vi "Edit_Raw_DF_Header.vi"(0 "Selected files":path[](array[path])) -> ()   [LabVIEW 2017]
uses:
  Controls/File_Selector_Type.ctl
panel:
  in  "Variable names to add by hand":string[](array[string])
  in  "Variable values to add by hand":string[](array[string])
  out "No of Unfound files":i32
  out "Unfound Files":path[](array[path])
  out "File Number":i32
  out "Current case":string
  out "Currently Editting":path
  out "Summary values":string[](array[string])
  in  "New Variable values":string[](array[string])
  in  "Setup Information":i32[](listbox)
  in  "Variable names to Edit":string[](array[string])
  in  "OK":bool
  out "No of Files":i32
  in  "Previous Choice":path
  in  "Search String":string
  in  "At Dialog Prompt for Editting Raw data files":T1
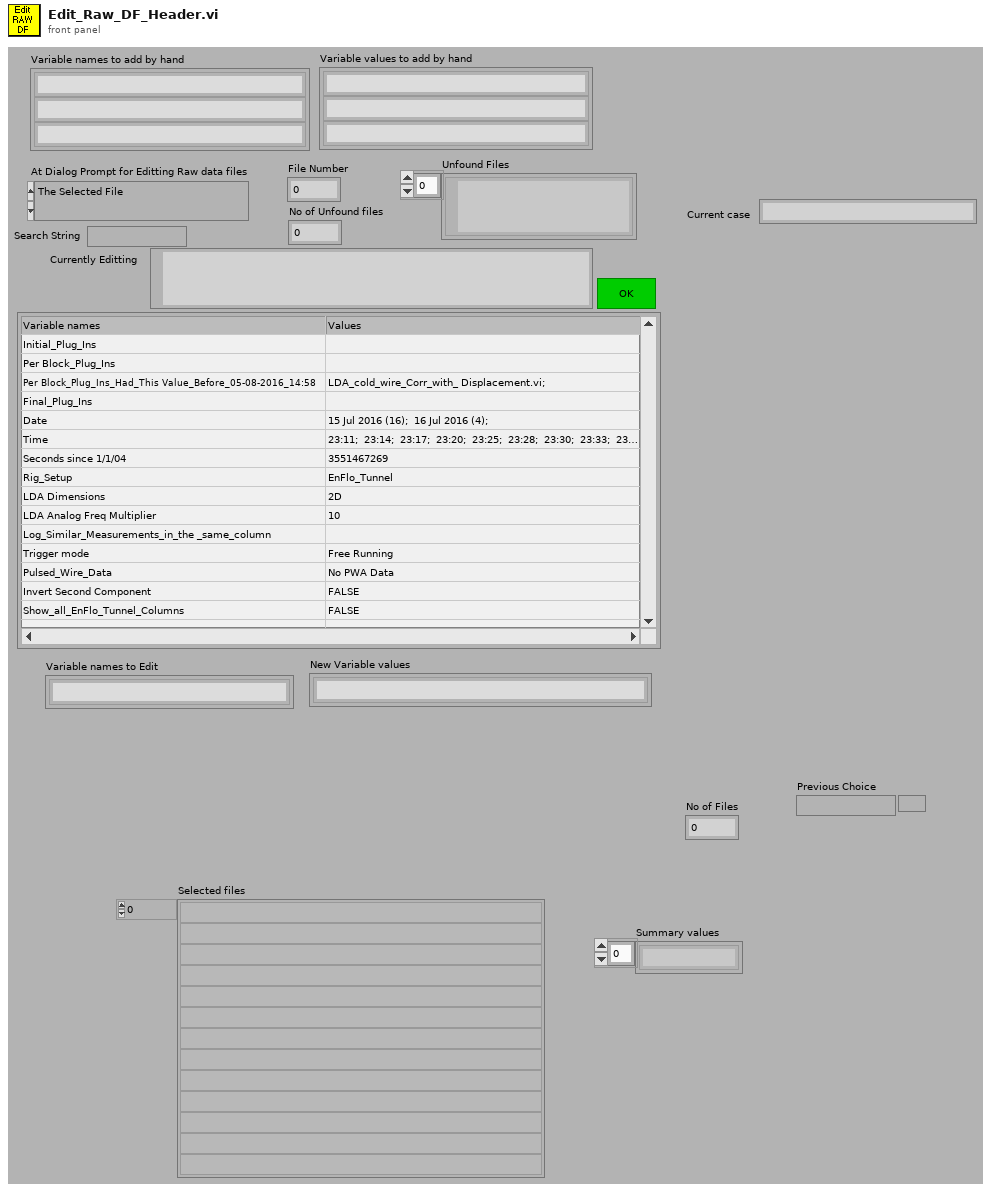
[diagram p1: front panel]
types:
  T1 = typedef "File_Selector_Type.ctl" = enum16{"The Selected File", "The Selected Folder", "Files containing the search string in the selected folder", "All files listed in selected file"}
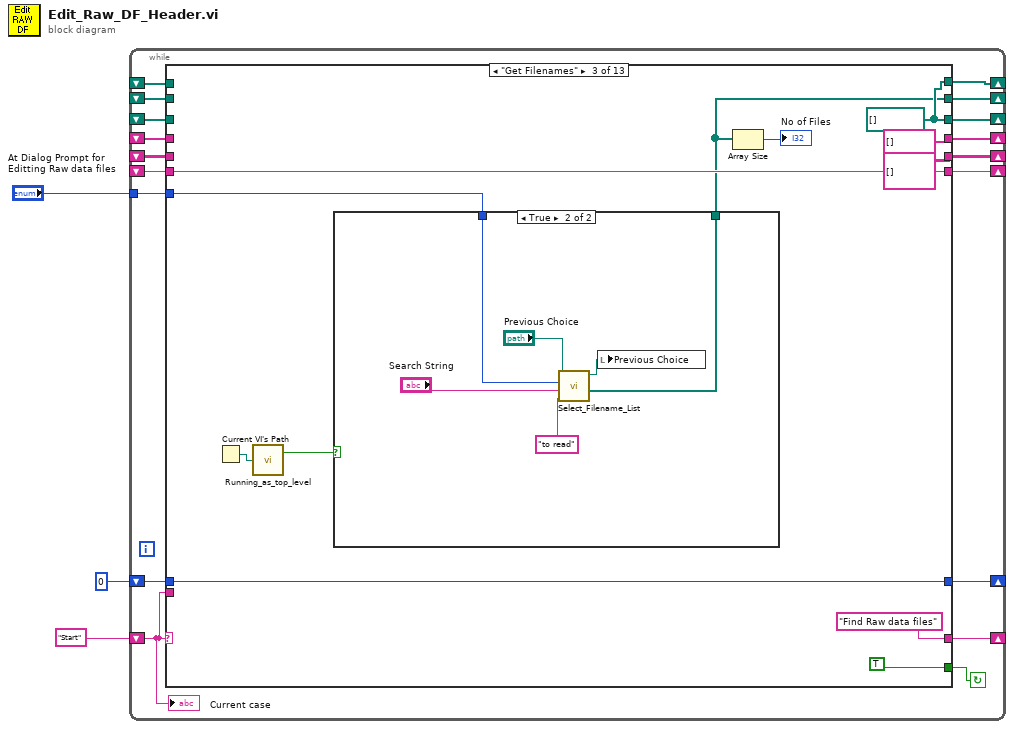
[diagram p0: block diagram]
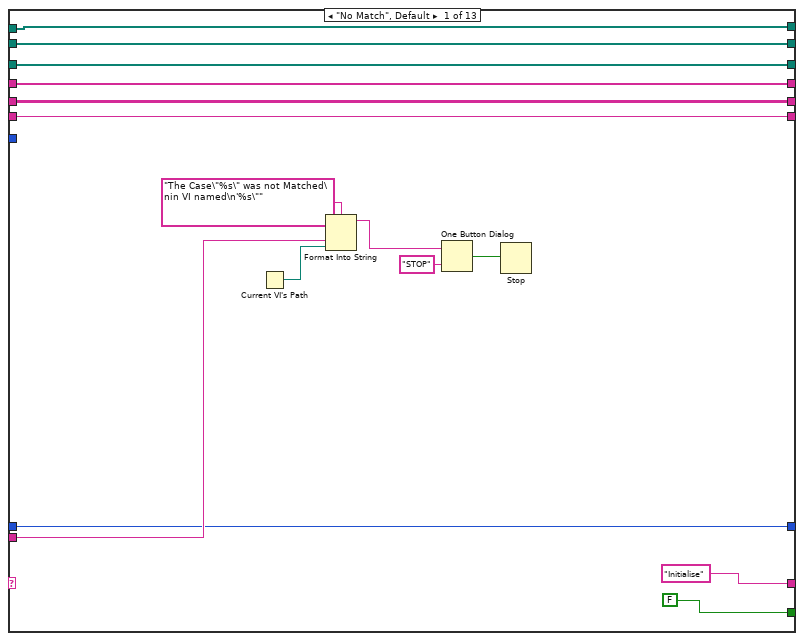
[diagram p2: hidden frame]
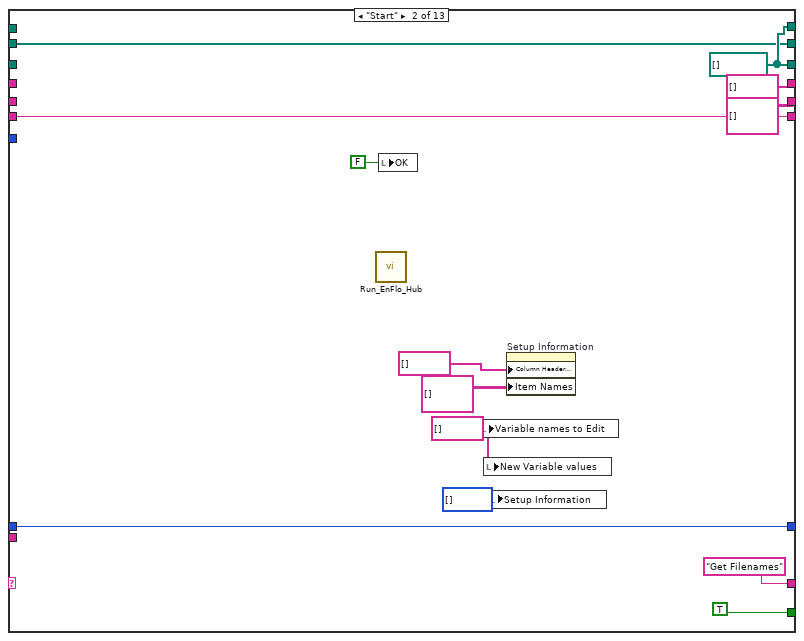
[diagram p3: hidden frame]
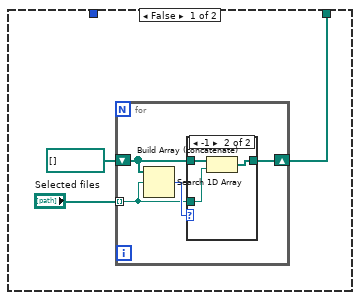
[diagram p4: hidden frame]
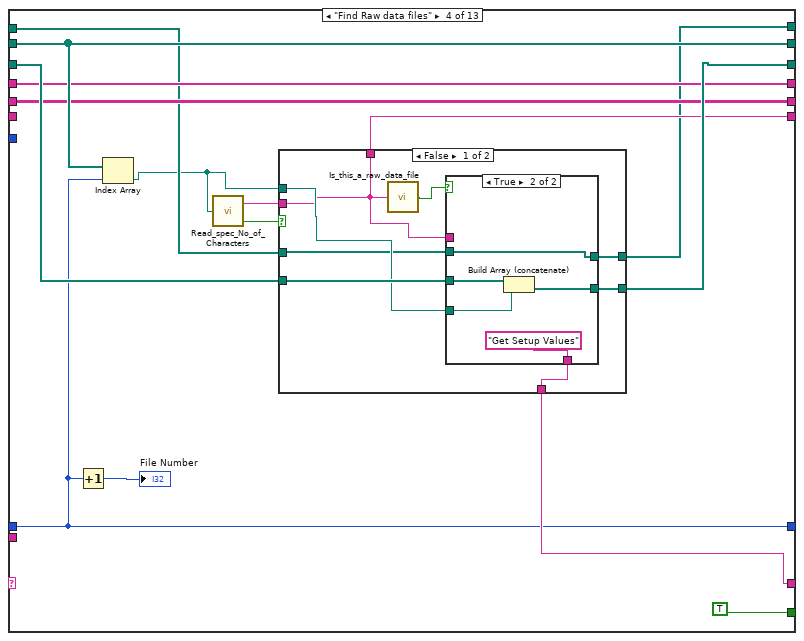
[diagram p6: hidden frame]
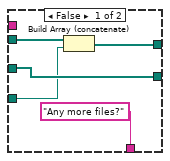
[diagram p7: hidden frame]
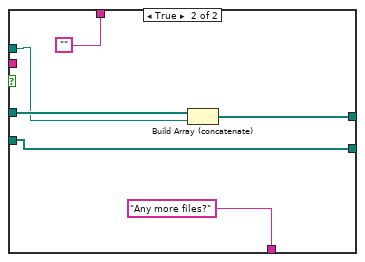
[diagram p8: hidden frame]
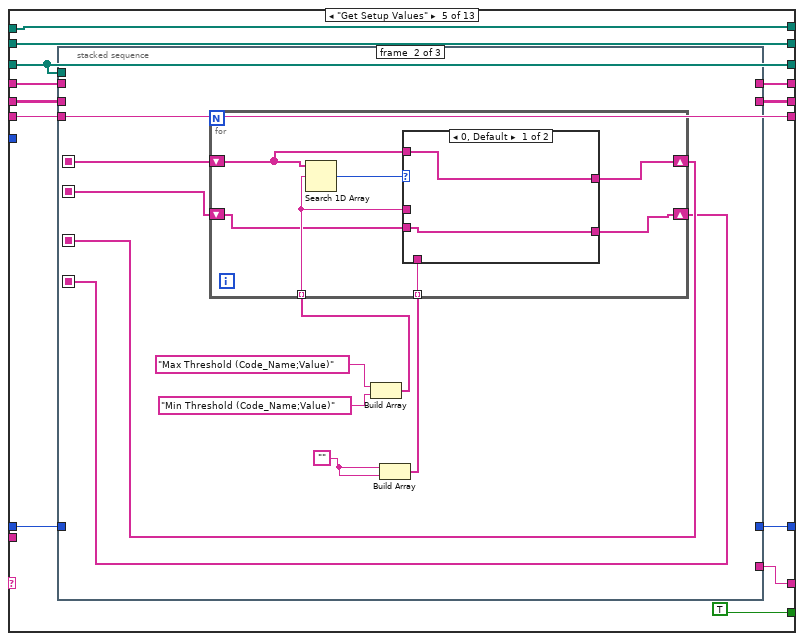
[diagram p9: hidden frame]
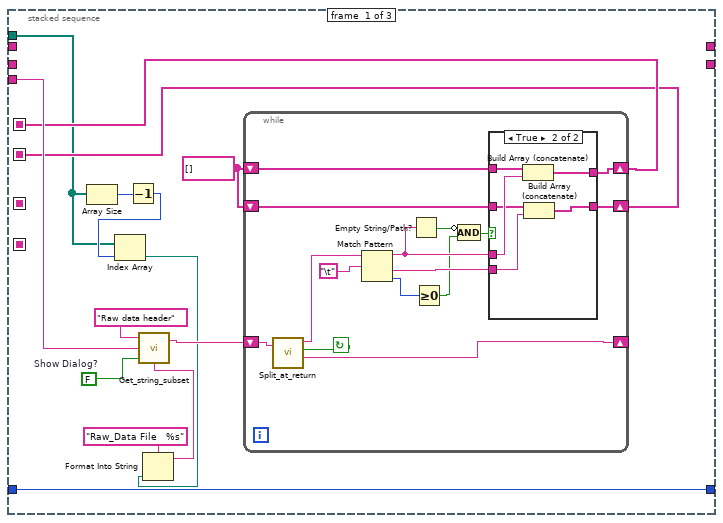
[diagram p10: hidden frame]
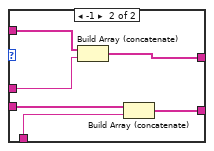
[diagram p12: hidden frame]
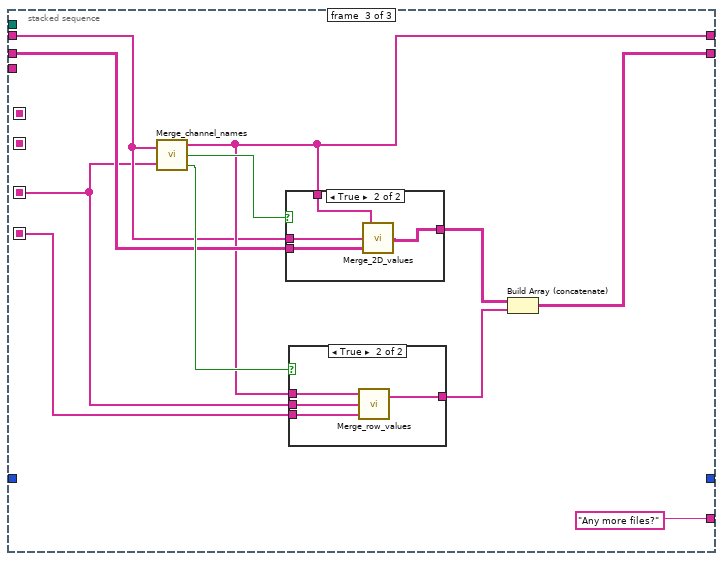
[diagram p13: hidden frame]
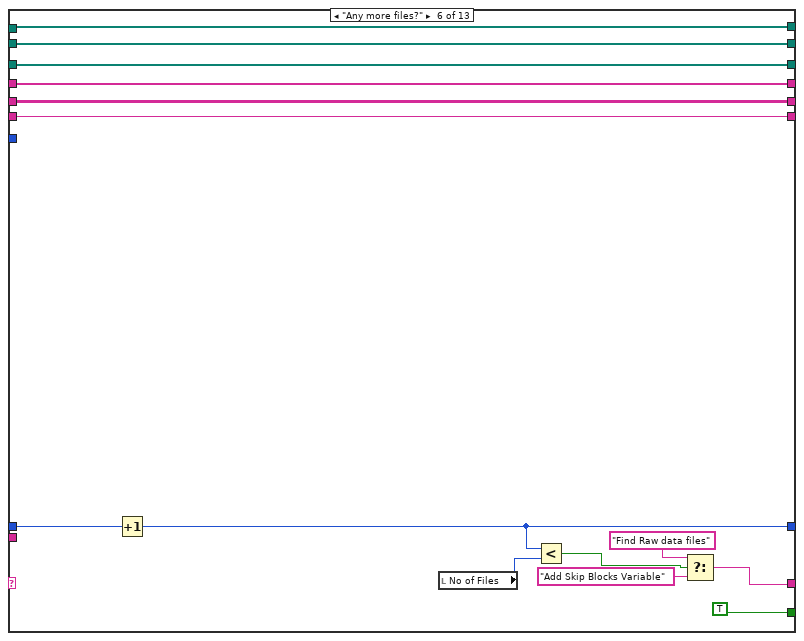
[diagram p16: hidden frame]
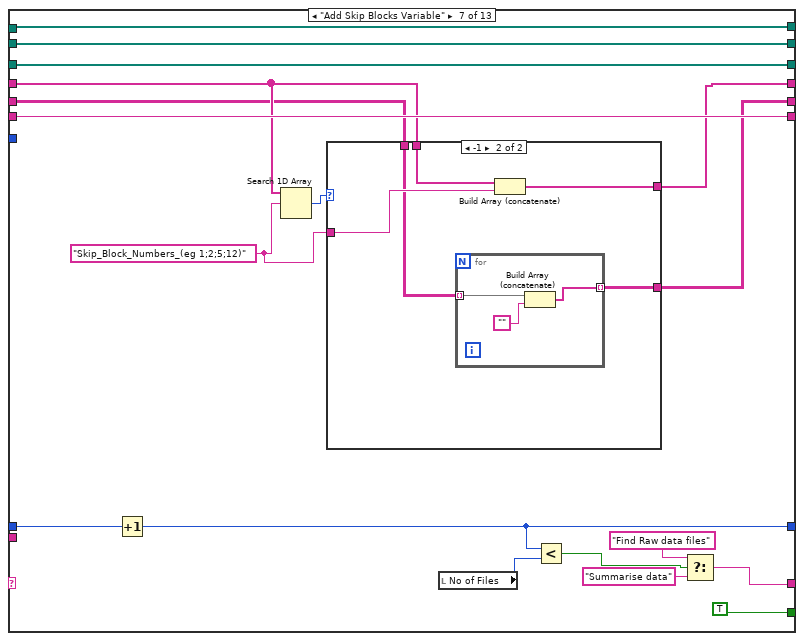
[diagram p17: hidden frame]
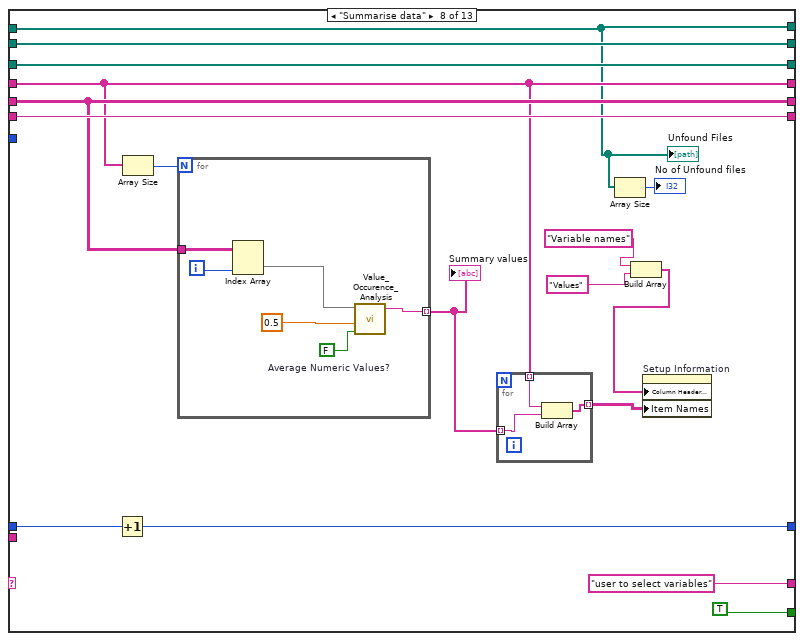
[diagram p19: hidden frame]
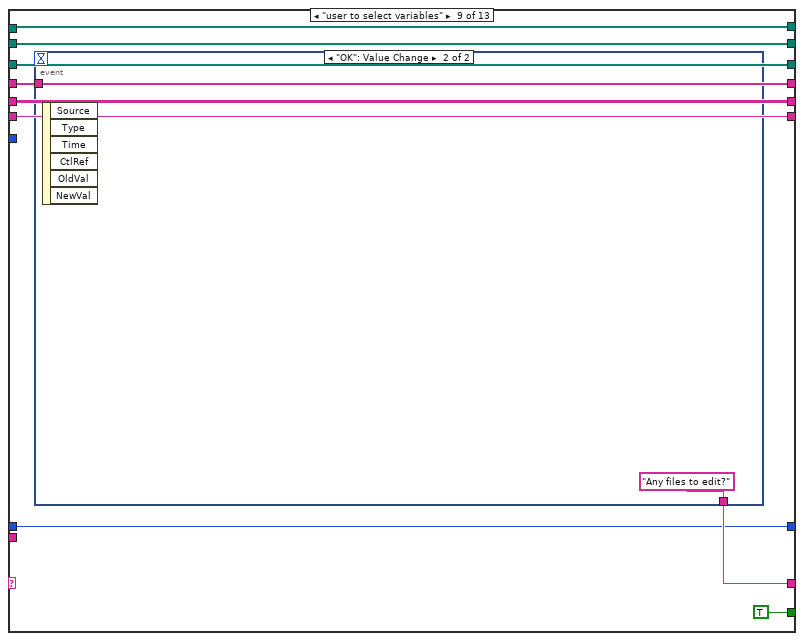
[diagram p20: hidden frame]
diagram:
  n1 = while {
    shift-left: "Start" -> [w19]
    shift-right: [w20] -> _
    shift-right: [w17] -> _
    shift-left: _ -> [w18]
    tunnel: "At Dialog Prompt for Editting Raw data files" -> [w16]
    shift-right: [w7] -> _
    shift-left: 0 -> [w13]
    shift-right: [w15] -> _
    shift-left: _ -> [w14]
    shift-right: [w12] -> _
    shift-left: _ -> [w11]
    shift-right: [w9] -> _
    shift-left: _ -> [w10]
    shift-right: [w8] -> _
    shift-left: _ -> [w6]
    shift-right: [w4] -> _
    shift-left: _ -> [w5]
    stop <- w21 continue-if-true
    n2 = case shown="\"Get Filenames\"" w19 {
      tunnel: [FALSE TRUE TRUE TRUE TRUE TRUE TRUE TRUE TRUE w323 w362 TRUE ("T button?") FALSE ("T button?")] -> w21
      tunnel: ["Initialise" "Get Filenames" "Find Raw data files" w86 w125 w217 w236 "user to select variables" w282 "Shall I edit the data files?" "Edit Raw data files" "End" "End"] -> w20
      tunnel: w19 -> [w31 _ _ _ _ _ _ _ _ _ _ _ _]
      tunnel: w18 -> [w28 w37 _ w90 w128 w224 w242 w269 w288 w336 w372 w383 w398]
      tunnel: [w28 w37 w50 w90 w128 w224 w242 w269 w288 w336 w372 w383 w398] -> w17
      tunnel: w16 -> [_ _ w60 _ _ _ _ _ _ _ _ _ _]
      tunnel: w14 -> [w27 _ _ w92 w118 w216 w235 w266 w287 w333 w366 w376 w392]
      tunnel: [w27 w38 w53 w91 w118 w216 w235 w266 w287 w333 w366 w376 w392] -> w15
      tunnel: w13 -> [w23 w44 w54 w85 w127 w222 w241 w268 w281 w335 w367 w378 w393]
      tunnel: [w26 string[] [] ("Merged Channels") string[] [] ("Merged Channels") w89 w123 w212 w230 w262 w283 w321 w369 w380 w395] -> w12
      tunnel: w11 -> [w26 _ _ w89 w120 w212 w231 w262 w283 w321 w369 w380 w395]
      tunnel: w10 -> [w25 _ _ w88 w122 w223 w227 w264 w285 w331 w370 w381 w396]
      tunnel: [w25 string[][] [] string[][] [] w88 w121 w223 w226 w264 w285 w331 w370 w381 w396] -> w9
      tunnel: [w24 w47 w57 w87 w124 w215 w234 w265 w286 w332 w371 w382 w397] -> w8
      tunnel: [w23 w44 w54 w85 w126 w221 w240 w267 w281 w334 w367 w378 w393] -> w7
      tunnel: w6 -> [w24 w47 w57 _ w124 w215 w234 w265 w286 w332 w371 w382 w397]
      tunnel: w5 -> [w22 _ _ w84 w119 w213 w232 w255 w280 w322 w361 w373 w388]
      tunnel: [w22 w38 w53 w83 w119 w213 w232 w255 w280 w322 w361 w373 w388] -> w4
      frame "No Match", Default {
        n3 = Current VI's Path() -> (path=w30:path)
        n4 = Format Into String(format string="The Case\"%s\" was not Matched\nin VI named\n'%s\"" ("Format String"), w31, w30) -> (resulting string=w34:string)  [unwired: 2 in, 1 out]
        n5 = One Button Dialog(message=w34, button name ("OK")="STOP") -> (true=w32:bool)
        n6 = Stop(stop? (T)=w32) -> ()
      }
      frame "Start" {
        w43 = string[] [] ("Variable names to Edit")
        w38 = path[] []
        n7 = call "Run_EnFlo_Hub.vi"() -> ()  [unwired: 1 in, 7 out]
        n8 = local write "OK"(FALSE ("OK")) -> ()
        n9 = local write "Variable names to Edit"(w43) -> ()
        n10 = local write "New Variable values"(w43) -> ()
        n11 = local write "Setup Information"(i32[] [] ("Setup Information")) -> ()
        n12 = property on="Setup Information" class="MCListbox (strict)"("Column Header Strings[]"=string[] [] ("Column Header Strings"), "Item Names"=string[][] []) -> ()  [unwired: 2 in, 2 out]
      }
      frame "Get Filenames" {
        w53 = path[] []
        n13 = Current VI's Path() -> (path=w52:path)
        n14 = call "Running_as_top_level.vi"("Vi path name"=w52) -> ("Top Level"=w51:bool)  [unwired: 1 out]
        n15 = case shown="True" w51 {
          tunnel: w60 -> [_ w78]
          tunnel: [w62 w73] -> w50
          frame False {
            n16 = for {
              shift-right: [w65] -> w62
              shift-left: path[] [] -> [w66]
              tunnel: "Selected files" -> [w67] mode=indexing
              n17 = Search 1D Array(1D array=w66, element=w67) -> (index of element=w68:i32)  [unwired: 1 in]
              n18 = case shown="-1" w68 {
                tunnel: w67 -> [_ w72]
                tunnel: w66 -> [w69 w71]
                tunnel: [w69 w70] -> w65
                frame Default {
                }
                frame -1 {
                  n19 = Build Array (concatenate)(w71, w72) -> (w70:path[])
                }
              }
            }
          }
          frame True {
            n20 = call "Select_Filename_List.vi"("File Type"="to read", "Search String"="Search String", "At Dialog Prompt Post Process"=w78, "Previous Choice"="Previous Choice") -> ("Selected files"=w73:path[], "Choosen path"=w74:path)  [unwired: 1 in, 2 out]
            n21 = local write "Previous Choice"(w74) -> ()
          }
        }
        n22 = Array Size(array=w50) -> (size(s)=→"No of Files":i32)
      }
      frame "Find Raw data files" {
        n23 = Increment(x=w85) -> (x+1=→"File Number":i32)
        n24 = Index Array(array=w90, index=w85) -> (element=w82:path)
        n25 = call "Read_spec_No_of_Characters.vi"("Filename"=w82) -> ("character string"=w80:string, "Error?"=w81:bool)
        n26 = case shown="False" w81 {
          tunnel: w92 -> [w101 w117]
          tunnel: [w100 w117] -> w91
          tunnel: w82 -> [w98 w113]
          tunnel: [w94 ""] -> w87
          tunnel: [w97 "Any more files?"] -> w86
          tunnel: w84 -> [w96 w114]
          tunnel: [w95 w112] -> w83
          tunnel: w80 -> [w94 _]
          frame False {
            n27 = call "Is_this_a_raw_data_file.vi"("character string"=w94) -> ("Raw Dat File?"=w99:bool)  [unwired: 2 out]
            n28 = case shown="True" w99 {
              tunnel: w101 -> [w106 w111]
              tunnel: w98 -> [w102 w110]
              tunnel: [w106 w109] -> w100
              tunnel: w94 -> [_ _]
              tunnel: ["Any more files?" "Get Setup Values"] -> w97
              tunnel: w96 -> [w104 w107]
              tunnel: [w103 w107] -> w95
              frame False {
                n29 = Build Array (concatenate)(w104, w102) -> (w103:path[])
              }
              frame True {
                n30 = Build Array (concatenate)(w111, w110) -> (w109:path[])
              }
            }
          }
          frame True {
            n31 = Build Array (concatenate)(w114, w113) -> (w112:path[])
          }
        }
      }
      frame "Get Setup Values" {
        n32 = stacked-sequence {
          seq-local: [w137 _ _] -> [_ w175 _]
          seq-local: [w136 _ _] -> [_ w171 _]
          seq-local: [_ w168 _] -> [_ _ w192]
          seq-local: [_ w167 _] -> [_ _ w191]
          tunnel: w127 -> [w140 _ _]
          tunnel: [w140 _ _] -> w126
          tunnel: [_ _ "Any more files?"] -> w125
          tunnel: w124 -> [w141 _ _]
          tunnel: w120 -> [_ _ w193]
          tunnel: [_ _ w195] -> w123
          tunnel: w122 -> [_ _ w199]
          tunnel: [_ _ w196] -> w121
          tunnel: w118 -> [w131 _ _]
          frame #0 {
            w138 = string[] []
            w143 = FALSE  # Show Dialog?
            n33 = Array Size(array=w131) -> (size(s)=w133:i32)
            n34 = Decrement(x=w133) -> (x-1=w132:i32)
            n35 = Index Array(array=w131, index=w132) -> (element=w130:path)
            n36 = Format Into String(format string="Raw_Data File   %s", w130) -> (resulting string=w134:string)  [unwired: 2 in, 1 out]
            n37 = call "Get_string_subset.vi"("String Name"=w134, "Show Dialog?"=w143, "String to split"=w141, "File Label"="Raw data header") -> ("Output string"=w139:string)  [unwired: 1 out]
            n38 = while {
              shift-right: [w157] -> _
              shift-left: w139 -> [w158]
              shift-right: [w151] -> w137
              shift-left: w138 -> [w152]
              shift-right: [w149] -> w136
              shift-left: w138 -> [w150]
              stop <- w156 continue-if-true
              n39 = call "Split_at_return.vi"("String"=w158) -> ("before substring"=w154:string, "Matched?"=w156:bool, "after substring"=w157:string)  [unwired: 1 in, 1 out]
              n40 = Match Pattern(string=w154, regular expression="\t") -> (before substring=w147:string, after substring=w148:string, offset past match=w153:i32)  [unwired: 2 out]
              n41 = Empty String/Path?(string/path=w147) -> (empty?=w146:bool)
              n42 = Greater Or Equal To 0?(x=w153) -> (x >= 0?=w144:bool)
              n43 = Compound Arithmetic op=AND(invert w146, w144) -> (w145:bool)
              n44 = case shown="True" w145 {
                tunnel: w152 -> [w160 w166]
                tunnel: w147 -> [_ w165]
                tunnel: [w160 w164] -> w151
                tunnel: w150 -> [w159 w163]
                tunnel: [w159 w162] -> w149
                tunnel: w148 -> [_ w161]
                frame False {
                }
                frame True {
                  n45 = Build Array (concatenate)(w166, w165) -> (w164:string[])
                  n46 = Build Array (concatenate)(w163, w161) -> (w162:string[])
                }
              }
            }
          }
          frame #1 {
            w169 = ""
            n47 = Build Array("Max Threshold (Code_Name;Value)", "Min Threshold (Code_Name;Value)") -> (w172:string[])
            n48 = Build Array(w169, w169) -> (w170:string[])
            n49 = for {
              shift-right: [w179] -> w168
              shift-left: w175 -> [w181]
              tunnel: w172 -> [w180] mode=indexing
              shift-right: [w176] -> w167
              shift-left: w171 -> [w178]
              tunnel: w170 -> [w177] mode=indexing
              n50 = Search 1D Array(1D array=w181, element=w180) -> (index of element=w182:i32)  [unwired: 1 in]
              n51 = case shown="0, Default" w182 {
                tunnel: w181 -> [w184 w190]
                tunnel: w180 -> [_ w189]
                tunnel: [w184 w188] -> w179
                tunnel: w178 -> [w183 w187]
                tunnel: w177 -> [_ w186]
                tunnel: [w183 w185] -> w176
                frame 0, Default {
                }
                frame -1 {
                  n52 = Build Array (concatenate)(w190, w189) -> (w188:string[])
                  n53 = Build Array (concatenate)(w187, w186) -> (w185:string[])
                }
              }
            }
          }
          frame #2 {
            n54 = call "Merge_channel_names.vi"("Preferred Channel array"=w193, "Channel array"=w192) -> ("Merged Channels"=w195:string[], "Preferred Channels Changed?"=w200:bool, "Channel Array Changed?"=w201:bool)
            n55 = case shown="True" w200 {
              tunnel: w199 -> [w207 w209]
              tunnel: w193 -> [_ w211]
              tunnel: [w207 w208] -> w198
              tunnel: w195 -> [_ w210]
              frame False {
              }
              frame True {
                n56 = call "Merge_2D_values.vi"("Values In"=w209, "Present Channels"=w211, "Desired Channels"=w210) -> ("Values Out"=w208:string[][])
              }
            }
            n57 = case shown="True" w201 {
              tunnel: [w202 w206] -> w197
              tunnel: w195 -> [_ w205]
              tunnel: w192 -> [_ w204]
              tunnel: w191 -> [w202 w203]
              frame False {
              }
              frame True {
                n58 = call "Merge_row_values.vi"("Present Row values"=w203, "Present Channels"=w204, "Desired Channels"=w205) -> ("Desired Row values"=w206:string[])  [unwired: 1 out]
              }
            }
            n59 = Build Array (concatenate)(w198, w197) -> (w196:string[][])
          }
        }
      }
      frame "Any more files?" {
        n60 = Increment(x=w222) -> (x+1=w221:i32)
        n61 = local read "No of Files"() -> (w220:i32)
        n62 = Less?(x=w221, y=w220) -> (x < y?=w219:bool)
        n63 = Select(t="Find Raw data files", s=w219, f="Add Skip Blocks Variable") -> (s? t:f=w217:string)
      }
      frame "Add Skip Blocks Variable" {
        w229 = "Skip_Block_Numbers_(eg 1;2;5;12)" ("Variable name")
        n64 = Increment(x=w241) -> (x+1=w240:i32)
        n65 = Search 1D Array(1D array=w231, element=w229) -> (index of element=w228:i32)  [unwired: 1 out]
        n66 = case shown="-1" w228 {
          tunnel: w231 -> [w245 w250]
          tunnel: w229 -> [_ w249]
          tunnel: [w245 w248] -> w230
          tunnel: w227 -> [w244 w247]
          tunnel: [w244 w246] -> w226
          frame 0, Default {
          }
          frame -1 {
            n67 = for {
              tunnel: w247 -> [w252] mode=indexing
              tunnel: [w251] -> w246 mode=indexing
              n68 = Build Array (concatenate)(w252, "") -> (w251:string[])
            }
            n69 = Build Array (concatenate)(w250, w249) -> (w248:string[])
          }
        }
        n70 = local read "No of Files"() -> (w239:i32)
        n71 = Less?(x=w240, y=w239) -> (x < y?=w238:bool)
        n72 = Select(t="Find Raw data files", s=w238, f="Summarise data") -> (s? t:f=w236:string)
      }
      frame "Summarise data" {
        n73 = Increment(x=w268) -> (x+1=w267:i32)
        n74 = Array Size(array=w262) -> (size(s)=w263:i32)
        n75 = for {
          N: w263 -> [_]
          tunnel: w264 -> [w278]
          tunnel: [w274] -> w261 mode=indexing
          i -> [w279]
          w275 = FALSE  # Average Numeric Values?
          n76 = Index Array(array=w278, index (col)=w279) -> (element=w277:string[])  [unwired: 1 in]
          n77 = call "Value_Occurence_Analysis.vi"("Average Numeric Values?"=w275, "Tolerance"=0.5, "String Array"=w277) -> ("Output String"=w274:string)  [unwired: 1 in, 2 out]
        }
        "Summary values" <- w261
        n78 = for {
          tunnel: w262 -> [w272] mode=indexing
          tunnel: w261 -> [w273] mode=indexing
          tunnel: [w271] -> w257 mode=indexing
          n79 = Build Array(w272, w273) -> (w271:string[])
        }
        n80 = Array Size(array=w255) -> (size(s)=→"No of Unfound files":i32)
        n81 = Build Array("Variable names", "Values") -> (w256:string[])
        n82 = property on="Setup Information" class="MCListbox (strict)"("Column Header Strings[]"=w256, "Item Names"=w257) -> ()  [unwired: 2 in, 2 out]
        "Unfound Files" <- w255
      }
      frame "user to select variables" {
        n83 = event shown="[1] \"OK\": Value Change" {
          selector: _ -> [_ _]
          dyn-events: _ -> [_ _]
          timeout: _ -> [_ _]
          tunnel: w283 -> [w297 _]
          tunnel: ["user to select variables" "Any files to edit?"] -> w282
          event "Setup Information": Value Change {
            n84 = event-data() -> ("NewVal"=w298:i32[])  [unwired: 6 out]
            n85 = local read "Summary values"() -> (w296:string[])
            n86 = for {
              tunnel: w298 -> [w304] mode=indexing
              tunnel: w297 -> [w307]
              tunnel: "Variable names to Edit" -> [w306]
              tunnel: [w305] -> w290 mode=indexing
              tunnel: w296 -> [w303]
              tunnel: [w302] -> w295 mode=indexing
              tunnel: "New Variable values" -> [w300]
              tunnel: [w299] -> w292
              i -> [w299]
              n87 = Index Array(array=w307, index=w304) -> (element=w305:string)
              n88 = Search 1D Array(1D array=w306, element=w305) -> (index of element=w301:i32)  [unwired: 1 out]
              n89 = case shown="-1" w301 {
                tunnel: w304 -> [_ w313]
                tunnel: w303 -> [_ w312]
                tunnel: [w308 w311] -> w302
                tunnel: w301 -> [w310 _]
                tunnel: w300 -> [w309 _]
                frame 0, Default {
                  n90 = Index Array(array=w309, index=w310) -> (element=w308:string)
                }
                frame -1 {
                  n91 = Index Array(array=w312, index=w313) -> (element=w311:string)
                }
              }
            }
            n92 = Increment(x=w292) -> (x+1=w291:i32)
            n93 = local write "New Variable values"(w295) -> ()
            n94 = local write "Variable names to Edit"(w290) -> ()
            n95 = property on="Variable names to Edit" class="Arr (strict)"("Number of Rows"=w291) -> ()  [unwired: 2 in, 2 out]
            n96 = property on="New Variable values" class="Arr (strict)"("Number of Rows"=w291) -> ()  [unwired: 2 in, 2 out]
          }
          event "OK": Value Change {
            n97 = event-data() -> ()  [unwired: 7 out]
          }
        }
      }
      frame "Any files to edit?" {
        w327 = string[] []
        n98 = local read "New Variable values"() -> (w320:string[])
        n99 = local read "Summary values"() -> (w328:string[])
        n100 = local read "Variable names to Edit"() -> (w317:string[])
        n101 = Increment(x=w335) -> (x+1=w334:i32)
        n102 = Build Array (concatenate)("Variable values to add by hand", w320) -> (w318:string[])
        n103 = Build Array (concatenate)("Variable names to add by hand", w317) -> (w315:string[])
        n104 = for {
          tunnel: "Setup Information" -> [w339]
          tunnel: w328 -> [w352]
          tunnel: w318 -> [w346] mode=indexing
          shift-right: [w349] -> w326
          shift-left: w327 -> [w350]
          shift-right: [w347] -> w325
          shift-left: w327 -> [w348]
          tunnel: w315 -> [w344] mode=indexing
          tunnel: w321 -> [w345]
          i -> [w338]
          n105 = Index Array(array=w339, index=w338) -> (element=w337:i32)
          n106 = Index Array(array=w345, index=w337) -> (element=w343:string)
          n107 = Index Array(array=w352, index=w337) -> (element=w351:string)
          n108 = Equal?(x=w351, y=w346) -> (x = y?=w342:bool)
          n109 = Equal?(x=w344, y=w343) -> (x = y?=w341:bool)
          n110 = And(x=w341, y=w342) -> (x .and. y?=w340:bool)
          n111 = case shown="False" w340 {
            tunnel: w350 -> [w358 w360]
            tunnel: [w357 w360] -> w349
            tunnel: w348 -> [w356 w359]
            tunnel: [w355 w359] -> w347
            tunnel: w346 -> [w354 _]
            tunnel: w344 -> [w353 _]
            frame False {
              n112 = Build Array (concatenate)(w356, w354) -> (w355:string[])
              n113 = Build Array (concatenate)(w358, w353) -> (w357:string[])
            }
            frame True {
            }
          }
        }
        n114 = local write "Variable names to Edit"(w326) -> ()
        n115 = local write "New Variable values"(w325) -> ()
        n116 = Array Size(array=w325) -> (size(s)=w324:i32)
        n117 = Greater Than 0?(x=w324) -> (x > 0?=w323:bool)
      }
      frame "Shall I edit the data files?" {
        n118 = Array Size(array=w366) -> (size(s)=w365:i32)
        n119 = Format Into String(format string="Do you want to edit these raw data header values in %d Raw Data Files?" ("message"), w365) -> (resulting string=w363:string)  [unwired: 2 in, 1 out]
        n120 = Two Button Dialog(message=w363) -> (T button?=w362:bool)  [unwired: 2 out]
        n121 = property on="Currently Editting" class="Path"("Visible"=w362) -> ()  [unwired: 2 in, 2 out]
      }
      frame "Edit Raw data files" {
        n122 = local read "Variable names to Edit"() -> (w377:string[])
        n123 = local read "New Variable values"() -> (w374:string[])
        n124 = for {
          tunnel: w377 -> [w387]
          tunnel: w374 -> [w384]
          tunnel: w376 -> [w385] mode=indexing
          w386 = TRUE  # Edit Raw Data Header Info
          n125 = call "Edit_Raw_DF_Remote.vi"("Edit Raw Data Header Info"=w386, "New Values In"=w384, "New Chs In"=w387, "Current Filename"=w385) -> ()  [unwired: 4 out]
          "Currently Editting" <- w385
        }
      }
      frame "End" {
        n126 = property on="Currently Editting" class="Path"("Visible"=FALSE) -> ()  [unwired: 2 in, 2 out]
        n127 = local write "OK"(FALSE ("OK")) -> ()
      }
    }
    "Current case" <- w19
  }
